vi "极性转换.vi"(1 "1、0码":u32[](array[numeric])) -> (0 "0、-1码":i32[](array[numeric]))   [LabVIEW 2013]
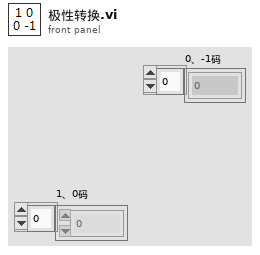
[diagram p1: front panel]
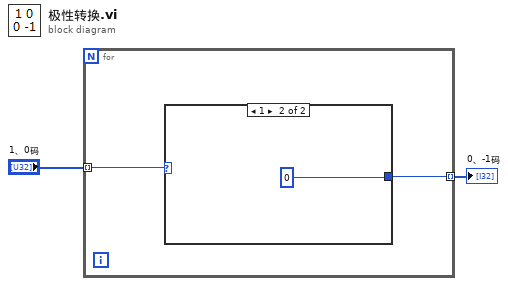
[diagram p0: block diagram]
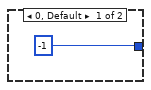
[diagram p2: hidden frame]
diagram:
  n1 = for {
    tunnel: "1、0码" -> [w4] mode=indexing
    tunnel: [w3] -> w1 mode=indexing
    n2 = case shown="1" w4 {
      tunnel: [-1 0] -> w3
      frame 0, Default {
      }
      frame 1 {
      }
    }
  }
  "0、-1码" <- w1
